vi "综合生物毒性_MB_api.vi"(5 "连接配置":T1={"连接类型"=enum."串口", "串口"="", "IP"="192.168.1.205", "PORT"="502"}, 7 "STEP":enum16{"open", "read", "write", "close"}(ring)=enum."read", 8 "Error in":errorcluster caption="Error in (no error)", 9 "values":u16, 10 "quantity":u16, 11 "starting address":u16 format="%04xH") -> (0 "error out":errorcluster, 1 "MB session out":refnum<class "MB_Master.lvclass">, 2 "输出簇":T2, 3 "Registers":u16[](array[numeric]))   [LabVIEW 2016, in "综合生物毒性.lvlib"]
uses:
  <vilib>/Plasmionique/MB Master/MB_Master/MB_Master.lvclass
  <vilib>/Plasmionique/MB Master/MB_ADU/MB_ADU.lvclass/MB_ADU.ctl
  <vilib>/Plasmionique/MB Master/MB_ADU/Read RX Data.vi
  <vilib>/Plasmionique/MB Master/MB_ADU/Read RX Timestamp.vi
  <vilib>/Plasmionique/MB Master/MB_ADU/Read Slave ID.vi
  <vilib>/Plasmionique/MB Master/MB_ADU/Read TX Data.vi
  <vilib>/Plasmionique/MB Master/MB_ADU/Read TX Timestamp.vi
  <vilib>/Plasmionique/MB Master/MB_Master_Serial/MB_Master_Serial.lvclass
  C:/Program Files (x86)/National Instruments/LabVIEW 2016/vi.lib/Plasmionique/MB Master/MB_Master/MB_Master.lvclass
  <vilib>/Plasmionique/MB Master/MB_Master_TCP/MB_Master_TCP.lvclass
  <vilib>/Plasmionique/MB Master/MB_ADU/MB_ADU.lvclass
  <vilib>/Plasmionique/MB Master/MB Master.lvlib
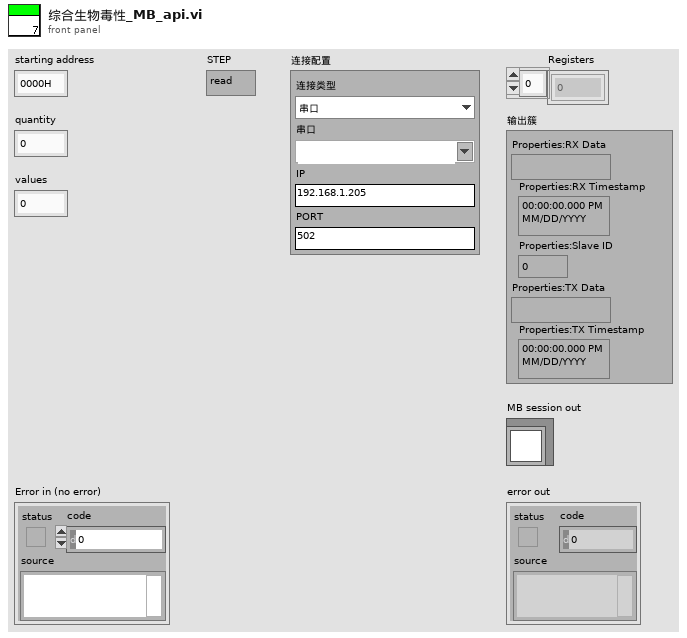
[diagram p1: front panel]
types:
  T1 = cluster{"连接类型":enum16{"串口", "TCP"}, "串口":string, "IP":string, "PORT":string}
  T2 = cluster{"Properties:RX Data":string, "Properties:RX Timestamp":timestamp, "Properties:Slave ID":u8, "Properties:TX Data":string, "Properties:TX Timestamp":timestamp}
  T3 = cluster{"baud rate (bps)":u32, "stop bits":u16, "parity":u16, "flow control":u16, "timeout":u32, "retries":i32}
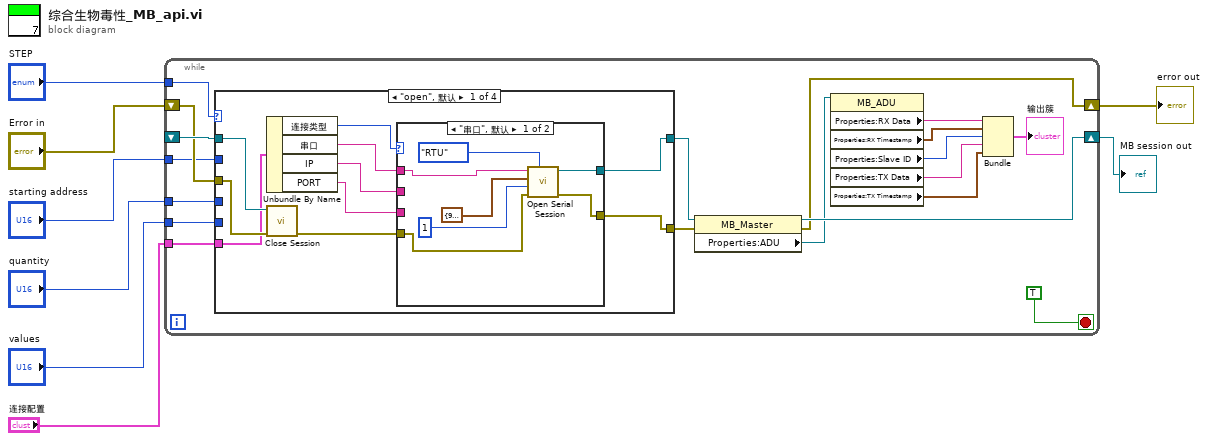
[diagram p0: block diagram]
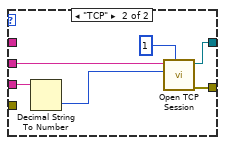
[diagram p2: hidden frame]
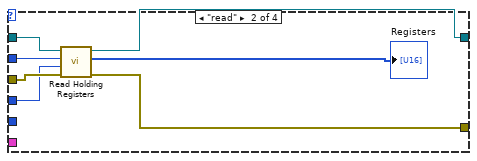
[diagram p3: hidden frame]
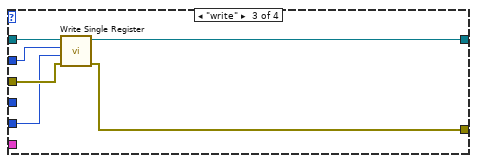
[diagram p4: hidden frame]
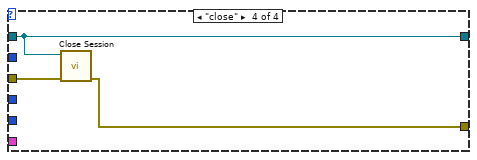
[diagram p5: hidden frame]
diagram:
  n1 = while {
    shift-right: [w21] -> w2
    shift-left: _ -> [w27]
    shift-right: [w19] -> w7
    shift-left: "Error in" -> [w26]
    tunnel: "starting address" -> [w25]
    tunnel: "quantity" -> [w24]
    tunnel: "STEP" -> [w23]
    tunnel: "values" -> [w12]
    tunnel: "连接配置" -> [w10]
    stop <- TRUE stop-if-true
    n2 = case shown="\"open\", 默认" w23 {
      tunnel: w27 -> [w35 w51 w61 w64]
      tunnel: w26 -> [w34 w57 w63 w66]
      tunnel: [w36 w56 w60 w64] -> w22
      tunnel: [w37 w55 w62 w65] -> w20
      tunnel: w25 -> [_ w53 w59 _]
      tunnel: w24 -> [_ w52 _ _]
      tunnel: w12 -> [_ _ w58 _]
      tunnel: w10 -> [w32 _ _ _]
      frame "open", Default {
        n3 = Unbundle By Name(w32) -> ("连接类型"=w31:enum16{"串口", "TCP"}, "串口"=w28:string, "IP"=w30:string, "PORT"=w29:string)
        n4 = call-dynamic "Close Session.vi"("error in (no error)"=w34, "MB session in"=w35) -> ("error out"=w33:errorcluster)  [unwired: 9 in]
        n5 = case shown="\"串口\", 默认" w31 {
          tunnel: [w42 w49] -> w37
          tunnel: [w40 w50] -> w36
          tunnel: w33 -> [w39 _]
          tunnel: w30 -> [_ w48]
          tunnel: w29 -> [_ w47]
          tunnel: w28 -> [w38 _]
          frame "串口", Default {
            n6 = call <vilib>:"Open Serial Session.vi"("Mode (RTU)"=enum16{"RTU", "ASCII"}."RTU", "Error in"=w39, "Slave ID"=u8 1, "Serial Config"=T3 {"baud rate (bps)"=9600, "stop bits"=10, "parity"=0, "flow control"=0, "timeout"=1000, "retries"=3}, "VISA Resource"=w38) -> ("Error out"=w42:errorcluster, "MB_Serial session"=w40:refnum<class "MB_Master_Serial.lvclass">)  [unwired: 5 in]
          }
          frame "TCP" {
            n7 = Decimal String To Number(string=w47) -> (number=w46:i32)  [unwired: 2 in, 1 out]
            n8 = call <vilib>:"Open TCP Session.vi"("Slave ID (255)"=u8 1, "Port (502)"=w46, "IP Address"=w48) -> ("error out"=w49:errorcluster, "MB_TCP session"=w50:refnum<class "MB_Master_TCP.lvclass">)  [unwired: 7 in]
          }
        }
      }
      frame "read" {
        n9 = call <vilib>:"Read Holding Registers.vi"("error in (no error)"=w57, "quantity"=w52, "starting address"=w53, "MB session in"=w51) -> ("error out"=w55:errorcluster, "Registers"=→"Registers":u16[], "MB session out"=w56:refnum<class "MB_Master.lvclass">)  [unwired: 5 in]
      }
      frame "write" {
        n10 = call <vilib>:"Write Single Register.vi"("error in (no error)"=w63, "value"=w58, "address"=w59, "MB session in"=w61) -> ("error out"=w62:errorcluster, "MB session out"=w60:refnum<class "MB_Master.lvclass">)  [unwired: 6 in]
      }
      frame "close" {
        n11 = call-dynamic "Close Session.vi"("error in (no error)"=w66, "MB session in"=w64) -> ("error out"=w65:errorcluster)  [unwired: 9 in]
      }
    }
    n12 = property class="MB_Master"(reference=w22, error in=w20) -> (reference out=w21:refnum<class "MB_Master.lvclass">, error out=w19:errorcluster, "Properties:ADU"=w9:refnum<class "MB_ADU.lvclass">)
    n13 = property class="MB_ADU"(reference=w9) -> ("Properties:RX Data"=w18:string, "Properties:RX Timestamp"=w17:timestamp, "Properties:Slave ID"=w16:u8, "Properties:TX Data"=w15:string, "Properties:TX Timestamp"=w14:timestamp)  [unwired: 1 in, 2 out]
    n14 = Bundle("Properties:RX Data"=w18, "Properties:RX Timestamp"=w17, "Properties:Slave ID"=w16, "Properties:TX Data"=w15, "Properties:TX Timestamp"=w14) -> (→"输出簇":T2)  [unwired: 1 in]
  }
  "error out" <- w7
  "MB session out" <- w2
